vi "Main.vi"() -> ()   [LabVIEW 2019]
doc: "This template is for the Queued Message Handler design pattern.\n\nThe Event Handling Loop generates messages based on user interface actions.\n\nThe Message Handling Loop processes messages generated by the Event Handling Loop, or by other messages. The messages are string values, so new messages can be added easily to the Message Cases case structure in the Message Handling Loop. Each message cluster can also provide an optional value for Message Data, which is a variant that can be converted to whatever message-specific data is required."
uses:
  controls/UI Data.ctl
  support/Message Queue/Enqueue Message (Single).vi
  GlobalVI.vi
  <vilib>/Instr/_visa.llb/VISA Configure Serial Port (Instr).vi
  <vilib>/Utility/error.llb/Error Cluster From Error Code.vi
  <vilib>/httpClient/POSTBuffer.vi
  <vilib>/ErrorRing/Error Ring.xnode
  <vilib>/regexp/Match Regular Expression.xnode
  support/Message Queue/Message Queue.lvlib
  support/User Event - Stop/User Event - Stop.lvlib
  <vilib>/httpClient/LabVIEWHTTPClient.lvlib
panel:
  in  "disconnectSerial":bool
  out "f":T1(ring)
  out "current time":timestamp format="%<%X\n%x>T"
  in  "disconnectSerial":bool
  in  "Tab Control":T2(tab)
  in  "E-mail":string
  in  "Name":string
  in  "UID":string
  in  "RequestHTTPLogout":bool
  out "authorized":bool
  in  "Password":string
  in  "Login":string
  in  "RequestHTTPLogin":bool
  in  "DeleteEmploye":bool
  in  "OK Button 2":bool
  in  "NewEmployee":bool
  in  "Hire date (dd/mm/yyyy hh:mm:ss)":string
  in  "Hourly Payment ($)":dbl
  in  "UID":string
  in  "E-mail":string
  in  "Name":string
  in  "Role":u16(ring) items=["Admin 1", "Admin 2", "Worker 1", "Worker 2"]
  in  "Hire Date":string
  out "Hourly Rate":dbl
  in  "Name":string
  in  "Check In":string
  in  "UID":string
  out "Role":u16(ring) items=["Admin 1", "Admin 2", "Worker 1", "Worker 2"]
  in  "Check In":string
  out "Work Hours":dbl
  in  "Hire Date":string
  out "Hourly Rate":dbl
  in  "Name":string
  in  "Check Out":string
  in  "UID":string
  out "Role":u16(ring) items=["Admin 1", "Admin 2", "Worker 1", "Worker 2"]
  out "buffer":string
  in  "Communication Port":refnum<visa-resource-name>
  out "Display <Replace Me>":string
  in  "connect":bool
  in  "Exit":bool
  # "Read Employee Info"
  # "put your card in our RFID\nreader to fill this field"
  # "put your card in our RFID\nreader to fill this field"
  # "put your card in our RFID\nreader to fill this field"
  # "put your card in our RFID\nreader to fill this field"
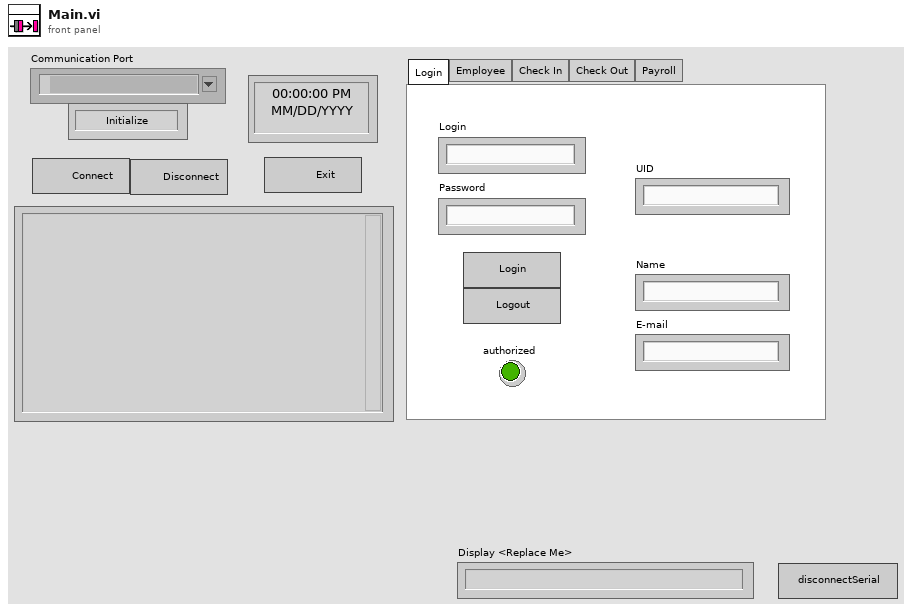
[diagram p1: front panel]
types:
  T1 = enum16{"Initialize", "Idle", "Connect", "Connected", "Disconnect", ""}
  T2 = enum32{"Login", "Employee", "Check In", "Check Out", "Payroll"}
  T3 = enum16{"Initialize", "Idle", "Connect", "Connected", "Disconnect"}
  T4 = typedef "UI Data.ctl" = cluster{"Boolean <Replace Me>":bool, "String <Replace Me>":string, "Numeric <Replace Me>":dbl, "Do Something Ref":refnum<vi>, "Do Something Else Ref":refnum<vi>, "Data Display Ref":refnum<vi>, "Exit Button Ref":refnum<vi>}
  T5 = typedef "LabVIEWHTTPClient.lvlib/ClientHandle.ctl" = refnum<k1>
  T6 = typedef "Message Queue.lvlib/All Message Queues.ctl" = cluster{"UI":refnum<queue>, "HTTP":refnum<queue>, "Serial":refnum<queue>}
  T7 = cluster{"name":string, "email":string, "uid":string, "hire_date":string, "hourly_rate":dbl, "job":cluster{"id":u8}}
  T8 = cluster{"id":u8, "checkIn":string, "checkOut":string, "work_hours":string, "employee":cluster{"id":u8, "name":string, "email":string, "uid":string, "hourly_rate":dbl, "hire_date":string, "job":cluster{"id":u8}, "createdAt":string}, "createdAt":string}
  T9 = cluster{"id":u8, "checkIn":string, "checkOut":string, "work_hours":dbl, "employee":cluster{"id":u8, "name":string, "email":string, "uid":string, "hourly_rate":dbl, "hire_date":string, "job":cluster{"id":u8}, "createdAt":string}, "createdAt":string}
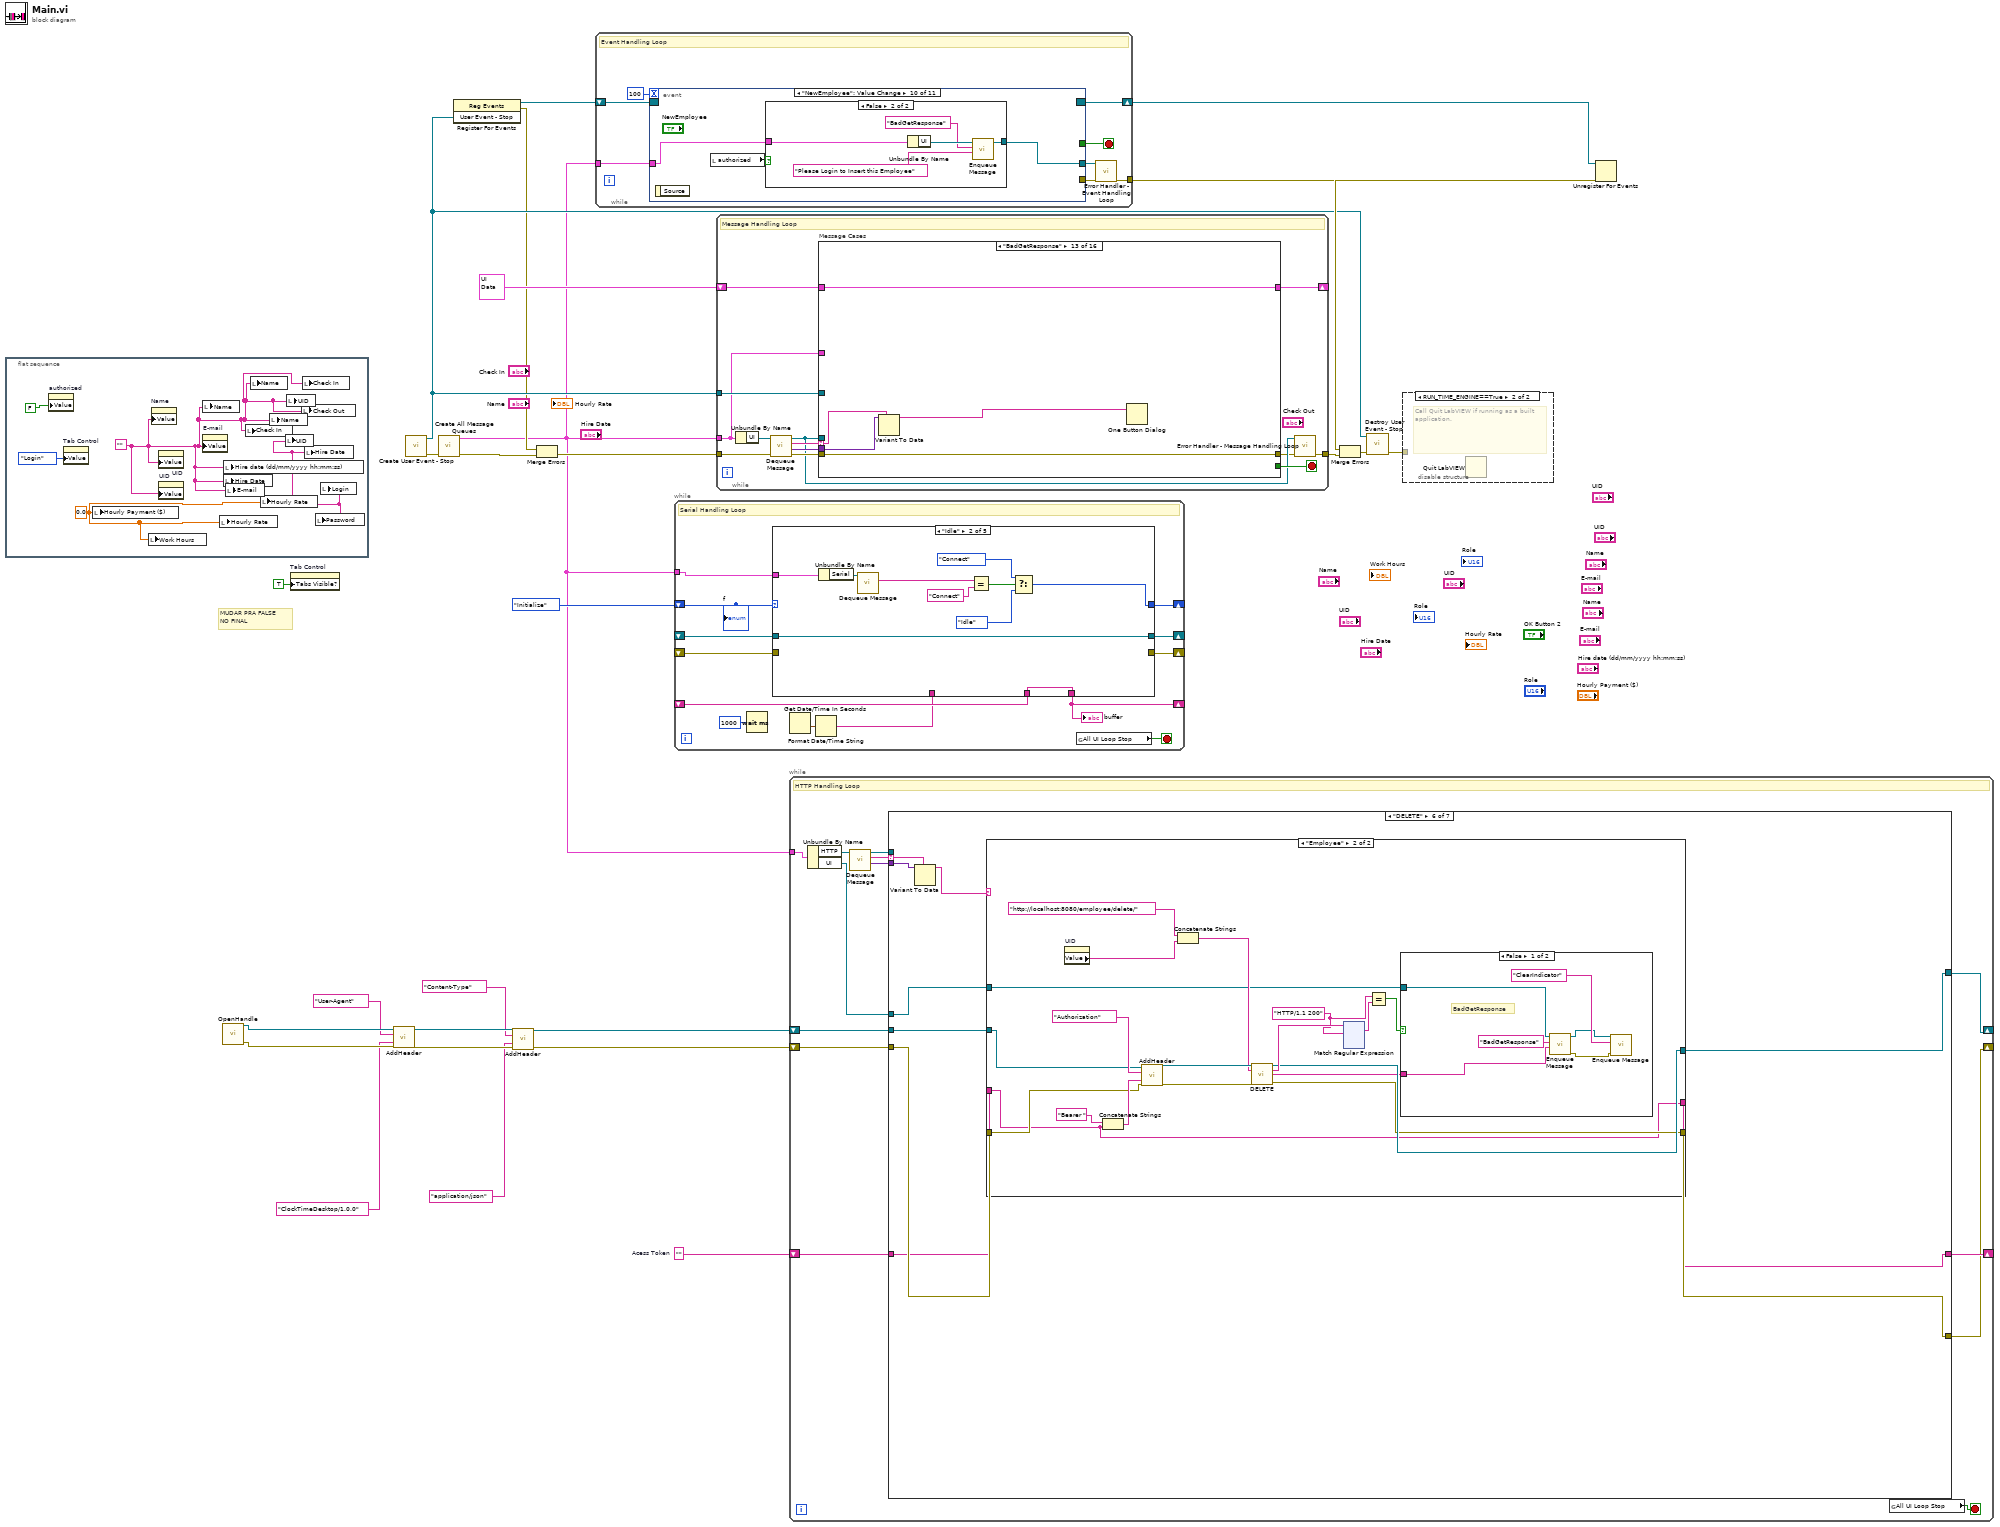
[diagram p0: block diagram]
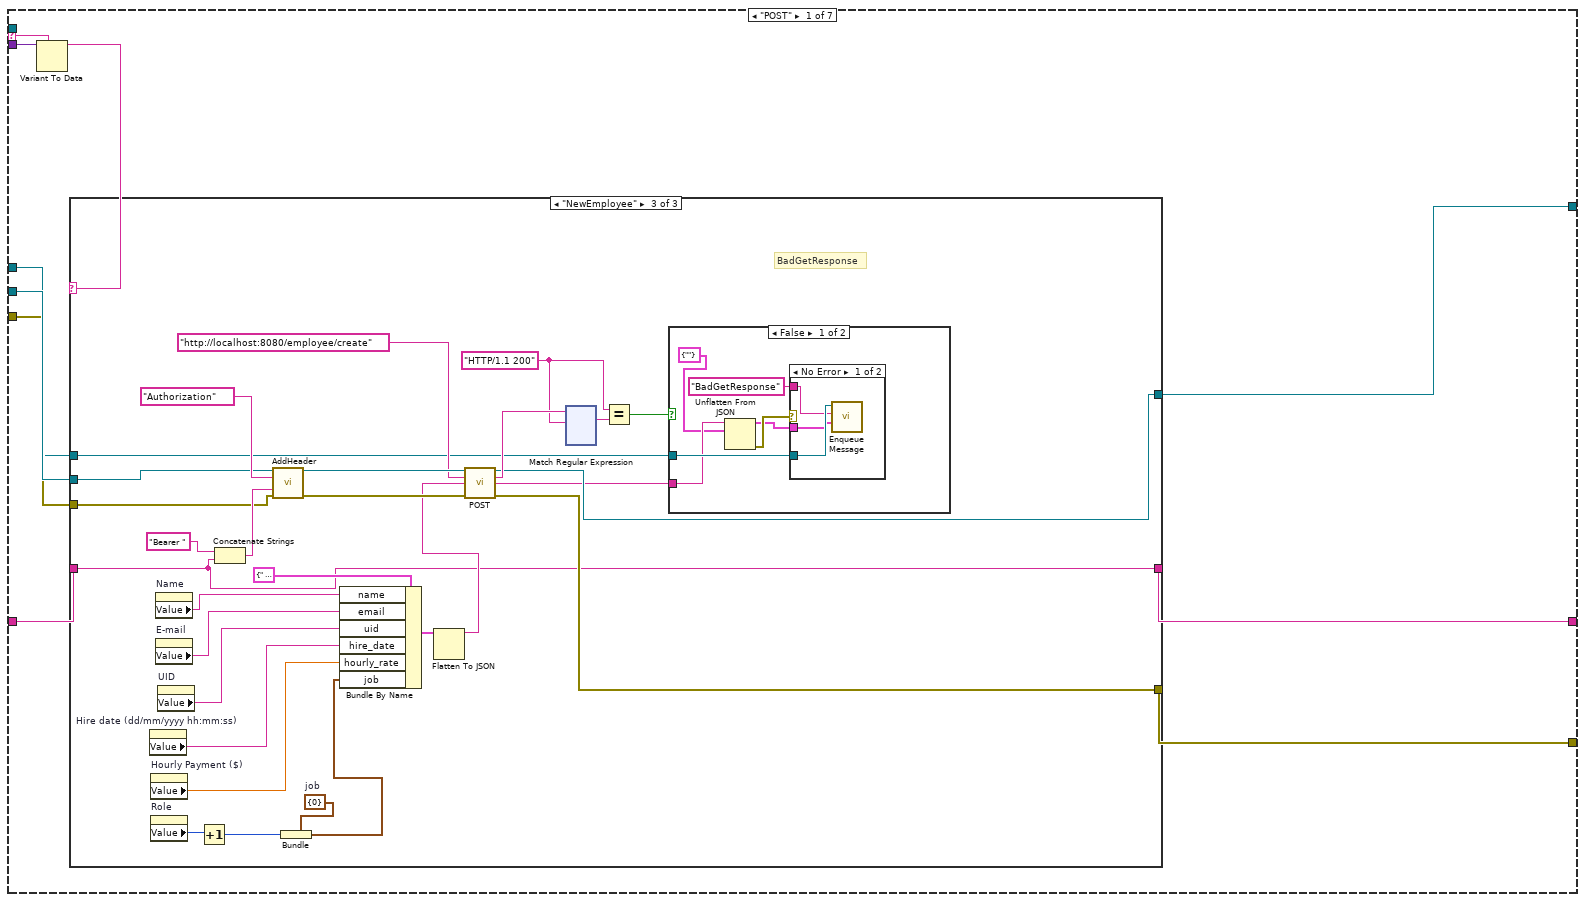
[diagram p2: hidden frame]
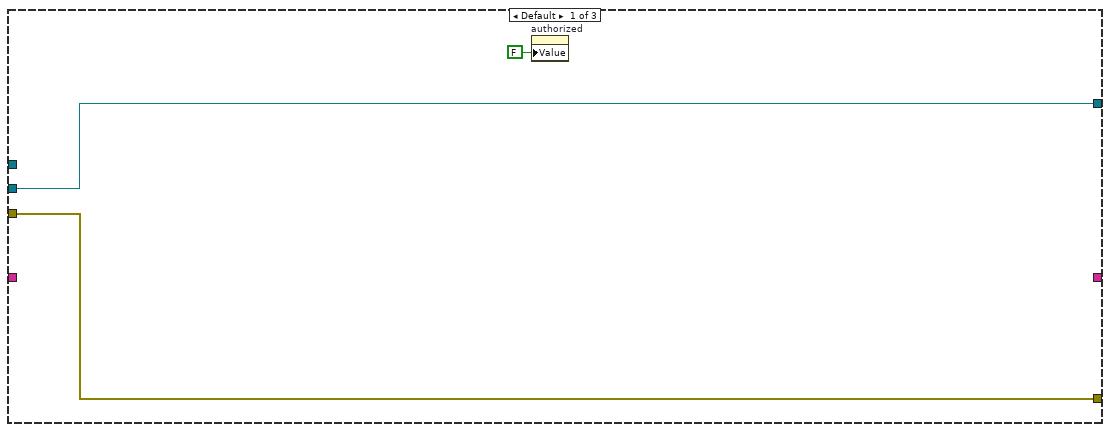
[diagram p3: hidden frame]
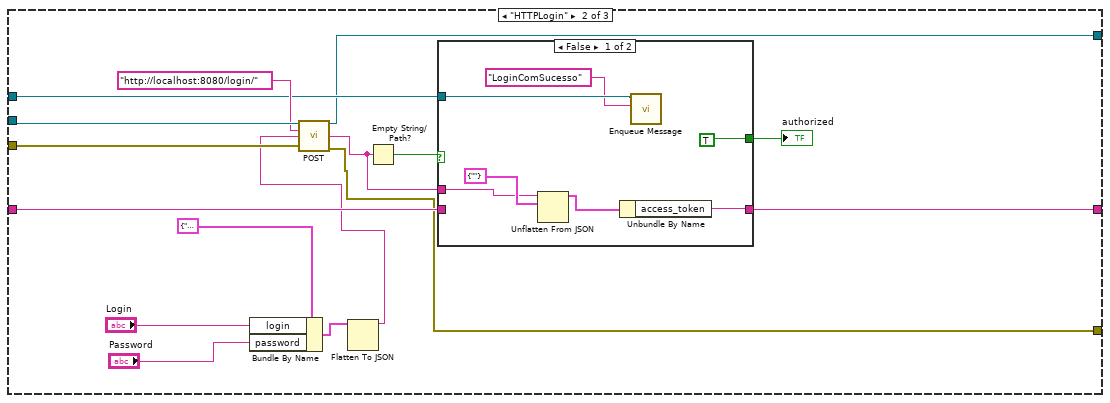
[diagram p4: hidden frame]
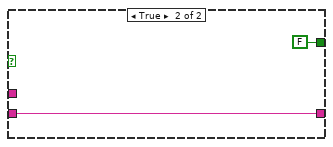
[diagram p5: hidden frame]
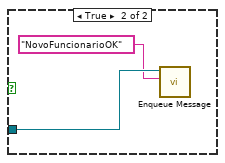
[diagram p7: hidden frame]
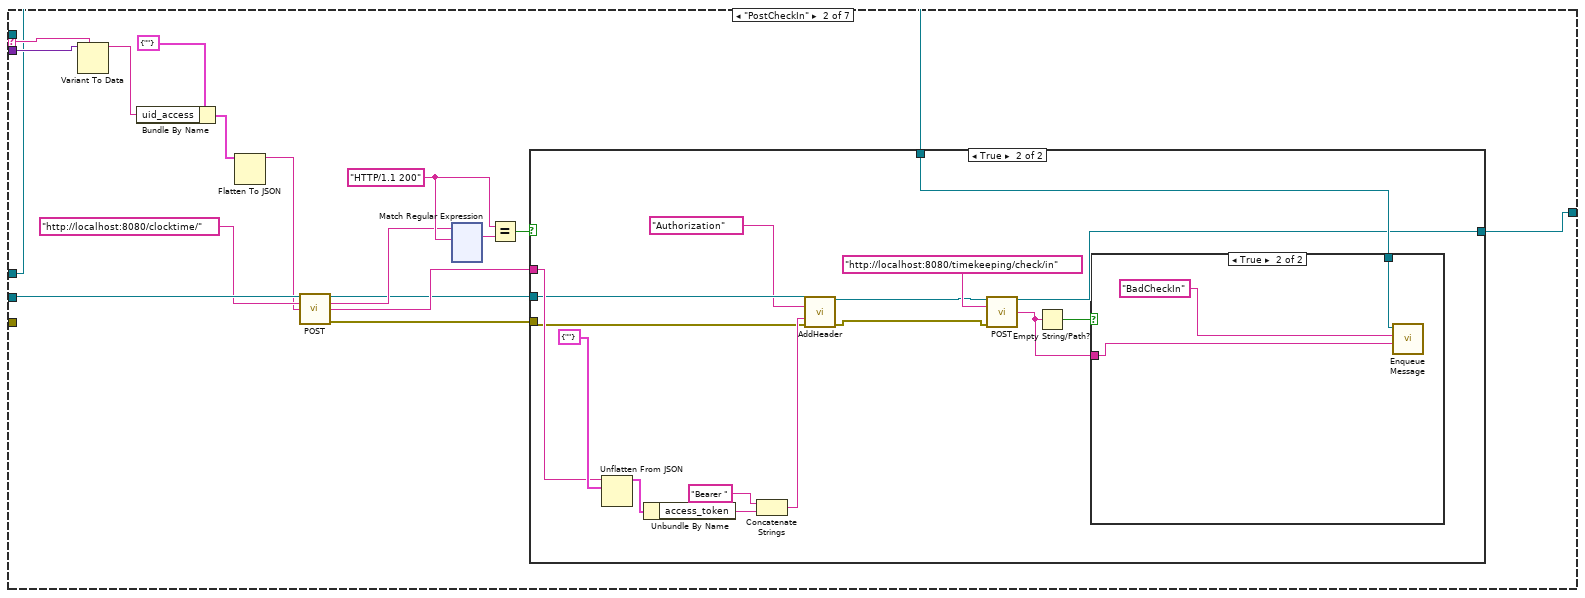
[diagram p8: hidden frame]
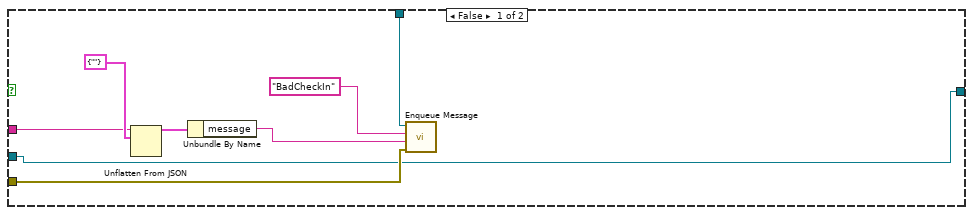
[diagram p9: hidden frame]
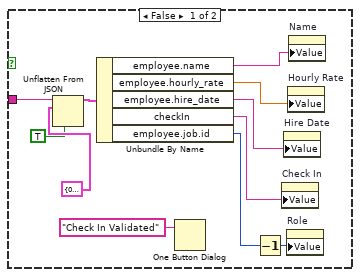
[diagram p10: hidden frame]
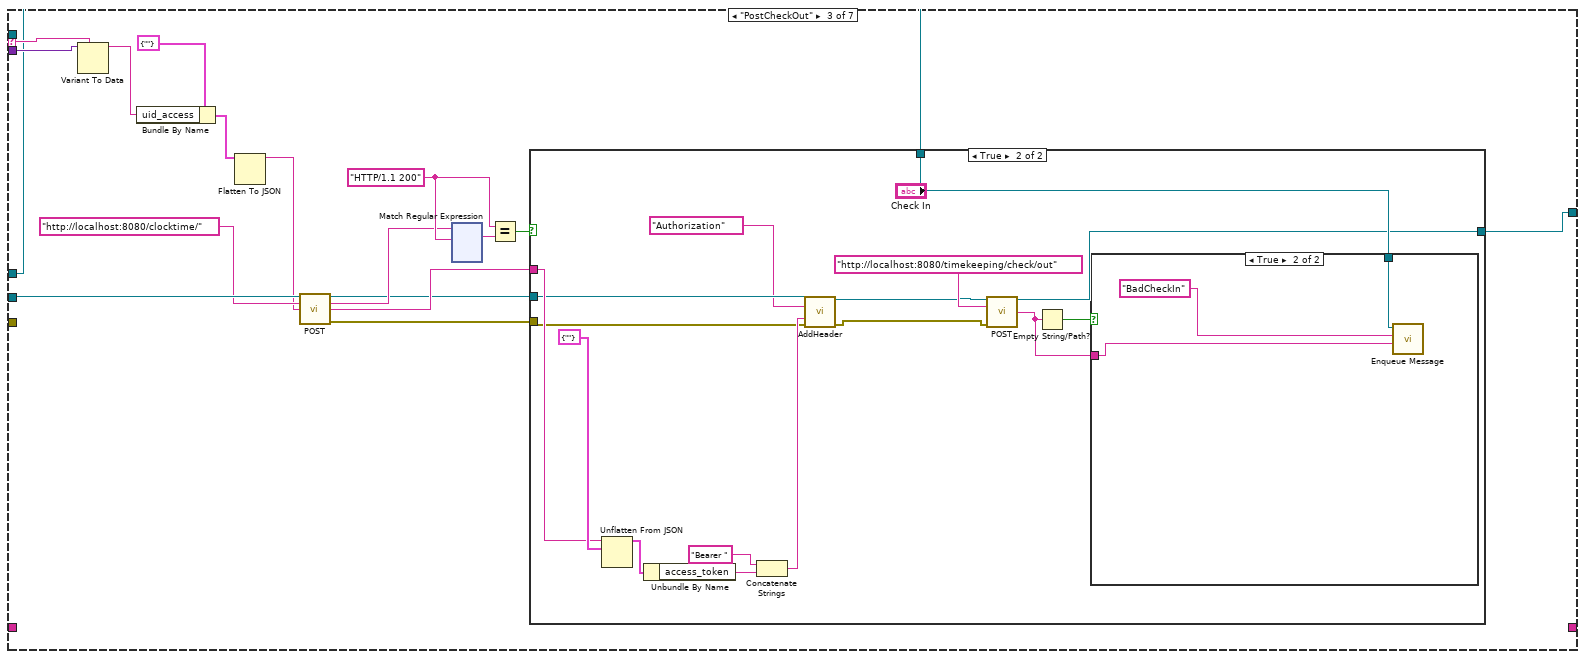
[diagram p11: hidden frame]
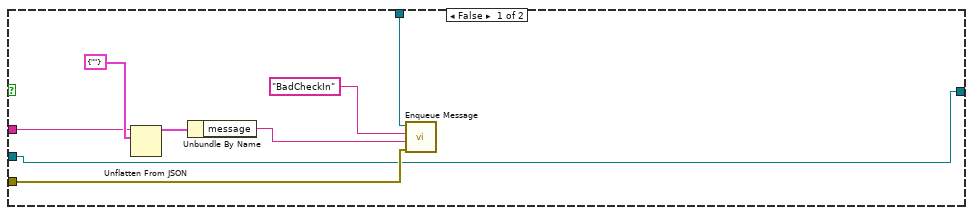
[diagram p12: hidden frame]
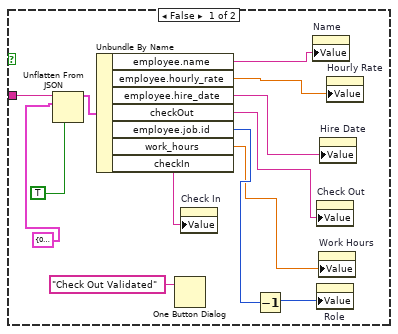
[diagram p13: hidden frame]
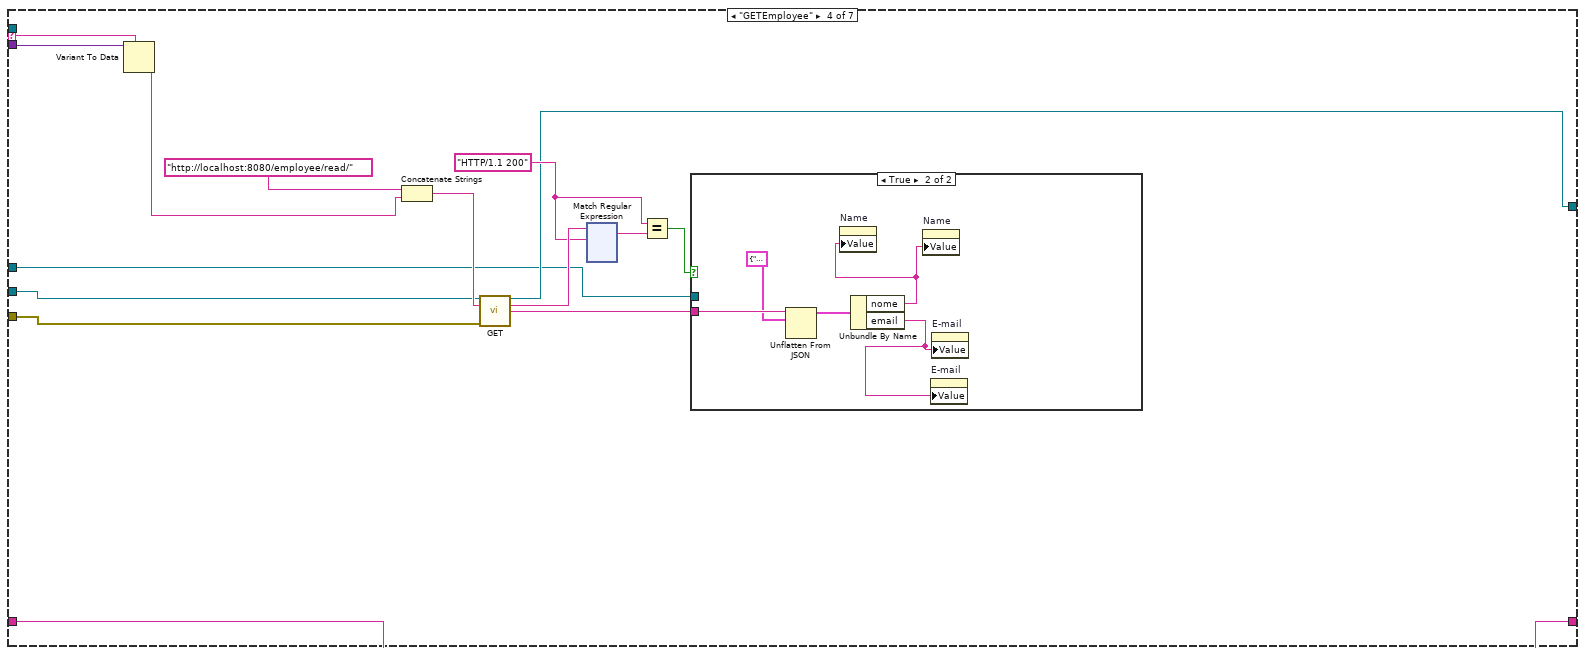
[diagram p14: hidden frame]
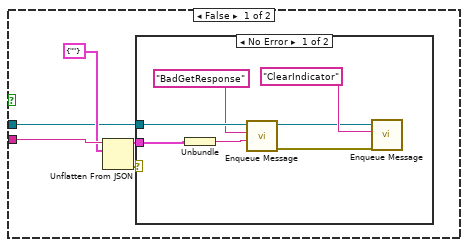
[diagram p15: hidden frame]
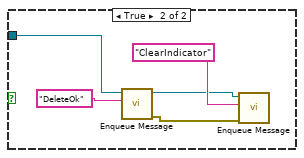
[diagram p19: hidden frame]
diagram:
  w12 = ""  # Acess Token
  # "MUDAR PRA FALSE \nNO FINAL"
  n1 = flat-sequence {
    frame #0 {
      w29 = 0.0 ("Hourly Payment ($)")
      w28 = ""
      n2 = property on="authorized" class="Bool (strict)"("Value"=FALSE ("authorized")) -> ()  [unwired: 2 in, 2 out]
      n3 = property on="Tab Control" class="TabCtl (strict)"("Value"=T2."Login" ("Tab Control")) -> ()  [unwired: 2 in, 2 out]
      n4 = local write "Hourly Payment ($)"(w29) -> ()
      n5 = local write "Work Hours"(w29) -> ()
      n6 = property on="Name" class="Str"("Value"=w28) -> ()  [unwired: 2 in, 2 out]
      n7 = property on="UID" class="Str"("Value"=w28) -> ()  [unwired: 2 in, 2 out]
      n8 = property on="UID" class="Str"("Value"=w28) -> ()  [unwired: 2 in, 2 out]
      n9 = local write "Name"(w28) -> ()
      n10 = property on="E-mail" class="Str"("Value"=w28) -> ()  [unwired: 2 in, 2 out]
      n11 = local write "Hourly Rate"(w29) -> ()
      n12 = local write "Hire date (dd/mm/yyyy hh:mm:ss)"(w28) -> ()
      n13 = local write "Hire Date"(w28) -> ()
      n14 = local write "E-mail"(w28) -> ()
      n15 = local write "Check In"(w28) -> ()
      n16 = local write "Name"(w28) -> ()
      n17 = local write "Hourly Rate"(w29) -> ()
      n18 = local write "Name"(w28) -> ()
      n19 = local write "UID"(w28) -> ()
      n20 = local write "UID"(w28) -> ()
      n21 = local write "Check Out"(w28) -> ()
      n22 = local write "Check In"(w28) -> ()
      n23 = local write "Hire Date"(w28) -> ()
      n24 = local write "Password"(w28) -> ()
      n25 = local write "Login"(w28) -> ()
    }
  }
  n26 = call <vilib>:"OpenHandle.vi"() -> ("client handle out"=w11:T5, "error out"=w9:errorcluster)  [unwired: 14 in]
  n27 = property on="Tab Control" class="TabCtl (strict)"("Tabs Visible?"=TRUE) -> ()  [unwired: 2 in, 2 out]
  n28 = call <vilib>:"AddHeader.vi"("client handle"=w11, "header"="User-Agent", "value"="ClockTimeDesktop/1.0.0", "error in (no error)"=w9) -> ("client handle out"=w10:T5, "error out"=w8:errorcluster)  [unwired: 10 in]
  n29 = call "Create User Event - Stop.vi"() -> ("error out"=w25:errorcluster, "User Event - Stop"=w17:refnum<user-event>)  [unwired: 10 in]
  n30 = call "Create All Message Queues.vi"("error in (no error)"=w25) -> ("error out"=w27:errorcluster, "Message Queues out"=w13:T6)  [unwired: 9 in]
  n31 = register-events(w17) -> (reference out=w18:refnum<event-registration>, error out=w15:errorcluster)  [unwired: 2 in]
  n32 = call <vilib>:"AddHeader.vi"("client handle"=w10, "header"="Content-Type", "value"="application/json", "error in (no error)"=w8) -> ("client handle out"=w7:T5, "error out"=w6:errorcluster)  [unwired: 10 in]
  n33 = Merge Errors(w15, w27) -> (w16:errorcluster)
  n34 = while {
    tunnel: w13 -> [w39]
    shift-right: [w37] -> w22
    shift-left: w18 -> [w38]
    tunnel: [w34] -> w19
    stop <- w35 stop-if-true
    # "Event Handling Loop"
    n35 = event shown="[9] \"NewEmployee\": Value Change" {
      selector: w38 -> [_ _ _ _ _ _ _ _ _ _ _]
      dyn-events: [_ _ _ _ _ _ _ _ _ _ _] -> w37
      timeout: 100 -> [_ _ _ _ _ _ _ _ _ _ _]
      tunnel: [_ _ _ _ _ _ _ TRUE ("Discard?") _ _ _] -> w35
      tunnel: w39 -> [w44 _ _ w52 w58 _ w62 _ w70 w75 w87]
      tunnel: [w42 _ _ w50 w57 _ w65 _ w71 _ w88] -> w36
      tunnel: [w40 _ _ w48 w53 _ w60 _ w72 w74 w89] -> w33
      event "connect": Value Change {
        n36 = event-data() -> ()  [unwired: 1 in, 1 out]
        n37 = Unbundle By Name(w44) -> ("Serial"=w41:refnum<queue>)
        n38 = call-poly "Enqueue Message.vi"("Message"="Connect", "Message Queue"=w41) -> ("error out"=w42:errorcluster, "dup Message Queue"=w40:refnum<queue>)  [unwired: 8 in]
      }
      event Timeout {
        n39 = event-data() -> ()  [unwired: 1 in, 1 out]
        n40 = Get Date/Time In Seconds() -> (seconds since 1Jan1904=→"current time":timestamp)
      }
      event "disconnectSerial": Value Change {
        n41 = event-data() -> ()  [unwired: 1 in, 1 out]
        n42 = property on="disconnectSerial" class="Bool (strict)"("Value"=TRUE ("disconnectSerial")) -> ()  [unwired: 2 in, 2 out]
      }
      event "RequestHTTPLogin": Value Change {
        n43 = event-data() -> ()  [unwired: 1 in, 1 out]
        n44 = Unbundle By Name(w52) -> ("HTTP"=w49:refnum<queue>)
        n45 = call-poly "Enqueue Message.vi"("Message Data"="HTTPLogin" ("Message"), "Message"="POST", "Message Queue"=w49) -> ("error out"=w50:errorcluster, "dup Message Queue"=w48:refnum<queue>)  [unwired: 7 in]
      }
      event Panel Close? {
        # "Send the 'Confirm Quit' message if the user closes the panel of the VI. Discard the event so the 'Confirm Quit' message has a chance to run."
        n46 = event-data() -> ()  [unwired: 1 in, 1 out]
        n47 = Unbundle By Name(w58) -> ("UI"=w54:refnum<queue>)
        n48 = call-poly "Enqueue Message.vi"("Priority Message? (F)"=TRUE, "Message"="Confirm Quit", "Message Queue"=w54) -> ("error out"=w57:errorcluster, "dup Message Queue"=w53:refnum<queue>)  [unwired: 7 in]
        n49 = event-data("Discard?"=TRUE) -> ()  [unwired: 1 in, 1 out]
      }
      event Application Instance Close {
        # "#CodeRecommended - When a project closes, all VIs within that project are aborted and leave memory. However, any code placed in this event frame is guaranteed to run to completion, so add any cleanup code that absolutely must happen here."
        n50 = event-data() -> ()  [unwired: 1 in, 1 out]
      }
      event "Exit": Value Change {
        n51 = event-data() -> ()  [unwired: 1 in, 1 out]
        n52 = Unbundle By Name(w62) -> ("UI"=w61:refnum<queue>)
        n53 = call-poly "Enqueue Message.vi"("Priority Message? (F)"=TRUE, "Message"="Exit", "Message Queue"=w61) -> ("error out"=w65:errorcluster, "dup Message Queue"=w60:refnum<queue>)  [unwired: 7 in]
      }
      event User Event {
        # "The Message Handling Loop processed an \"Exit\" message, which fired this event to stop the Event Handling Loop."
        n54 = event-data() -> ()  [unwired: 1 in, 1 out]
        n55 = local write "Display <Replace Me>"("\"Exit\" button pressed" ("VI Stopped")) -> ()
      }
      event "RequestHTTPLogout": Value Change {
        n56 = event-data() -> ()  [unwired: 1 in, 1 out]
        n57 = Unbundle By Name(w70) -> ("HTTP"=w69:refnum<queue>)
        n58 = call-poly "Enqueue Message.vi"("Message"="POST", "Message Queue"=w69) -> ("error out"=w71:errorcluster, "dup Message Queue"=w72:refnum<queue>)  [unwired: 8 in]
      }
      event "NewEmployee": Value Change {
        n59 = event-data() -> ()  [unwired: 1 in, 1 out]
        n60 = local read "authorized"() -> (w73:bool)
        n61 = case shown="False" w73 {
          tunnel: w75 -> [w80 w85]
          tunnel: [w76 w81] -> w74
          frame True {
            n62 = Unbundle By Name(w80) -> ("HTTP"=w79:refnum<queue>)
            n63 = call-poly "Enqueue Message.vi"("Message Data"="NewEmployee" ("Message"), "Message"="POST", "Message Queue"=w79) -> ("dup Message Queue"=w76:refnum<queue>)  [unwired: 7 in, 1 out]
          }
          frame False {
            n64 = Unbundle By Name(w85) -> ("UI"=w84:refnum<queue>)
            n65 = call-poly "Enqueue Message.vi"("Message Data"="Please Login to Insert this Employee" ("Message"), "Message"="BadGetResponse", "Message Queue"=w84) -> ("dup Message Queue"=w81:refnum<queue>)  [unwired: 7 in, 1 out]
          }
        }
      }
      event "DeleteEmploye": Value Change {
        n66 = event-data() -> ()  [unwired: 1 in, 1 out]
        n67 = local read "authorized"() -> (w86:bool)
        n68 = case shown="False" w86 {
          tunnel: [w95 w101] -> w89
          tunnel: [w94 w100] -> w88
          tunnel: w87 -> [w93 w99]
          frame True {
            n69 = Unbundle By Name(w93) -> ("HTTP"=w92:refnum<queue>)
            n70 = call-poly "Enqueue Message.vi"("Message Data"="Employee" ("Message"), "Message"="DELETE", "Message Queue"=w92) -> ("error out"=w94:errorcluster, "dup Message Queue"=w95:refnum<queue>)  [unwired: 7 in]
          }
          frame False {
            n71 = Unbundle By Name(w99) -> ("UI"=w98:refnum<queue>)
            n72 = call-poly "Enqueue Message.vi"("Message Data"="Please Login to delete this employee" ("Message"), "Message"="BadGetResponse", "Message Queue"=w98) -> ("error out"=w100:errorcluster, "dup Message Queue"=w101:refnum<queue>)  [unwired: 7 in]
          }
        }
      }
    }
    n73 = call "Error Handler - Event Handling Loop.vi"("error in (no error)"=w36, "Message Queue"=w33) -> ("dup error in"=w34:errorcluster)  [unwired: 8 in, 1 out]
  }
  n74 = while {
    tunnel: w13 -> [w111]
    shift-right: [w112] -> _
    shift-left: T3."Initialize" -> [w113]
    shift-right: [w110] -> _
    shift-left: _ -> [w108]
    shift-right: [w109] -> _
    shift-left: _ -> [w107]
    shift-right: [w105] -> _
    shift-left: _ -> [w106]
    stop <- w114 stop-if-true
    # "Serial Handling Loop"
    n75 = Wait (ms)(milliseconds to wait=u32 1000) -> ()  [unwired: 1 out]
    n76 = Get Date/Time In Seconds() -> (seconds since 1Jan1904=w104:timestamp)
    n77 = Format Date/Time String(seconds (now)=w104) -> (date/time string=w103:string)  [unwired: 2 in]
    n78 = case shown="\"Idle\"" w113 {
      tunnel: [T1."Idle" w118 w133 w142 _] -> w112
      tunnel: w111 -> [_ w124 _ w145 _]
      tunnel: [_ w117 w135 w143 _] -> w110
      tunnel: [_ _ w134 w144 w180] -> w109
      tunnel: w108 -> [_ w117 _ w149 w182]
      tunnel: w107 -> [_ _ _ w141 w181]
      tunnel: w106 -> [_ w116 w127 w139 w172]
      tunnel: [_ w116 w130 w138 w177] -> w105
      tunnel: w103 -> [_ _ w129 w137 w175]
      frame "Initialize", Default {
      }
      frame "Idle" {
        n79 = Unbundle By Name(w124) -> ("Serial"=w125:refnum<queue>)
        n80 = call "Dequeue Message.vi"("Message Queue"=w125) -> ("Message"=w123:string)  [unwired: 7 in, 3 out]
        n81 = Equal?(x=w123, y="Connect") -> (x = y?=w121:bool)
        n82 = Select(t=T1."Connect", s=w121, f=T1."Idle") -> (s? t:f=w118:T1)
      }
      frame "Connect" {
        n83 = call-poly "VISA Configure Serial Port"("VISA resource name"="Communication Port") -> ("VISA resource name out"=w135:refnum<visa-resource-name>, "error out"=w134:errorcluster)  [unwired: 13 in]
        n84 = Concatenate Strings("\r\n", w129, " - Connect" ("string"), w127) -> (w130:string)
        n85 = Select(t=T1."Idle" ("f"), s=w134, f=T1."Connected") -> (s? t:f=w133:T1)
      }
      frame "Connected" {
        n86 = property class="Instr"(reference=w149, error in=w141) -> (reference out=w147:refnum<visa-resource-name>, error out=w146:errorcluster, "Bytes at Port"=w140:u32)
        n87 = Greater Than 0?(x=w140) -> (x > 0?=w148:bool)
        n88 = case shown="True" w148 {
          tunnel: w147 -> [w157 w171]
          tunnel: w146 -> [w156 w170]
          tunnel: w145 -> [_ w169]
          tunnel: [w156 w166] -> w144
          tunnel: [w157 w165] -> w143
          tunnel: [w150 T1."Connected"] -> w142
          tunnel: w140 -> [_ w163]
          tunnel: w139 -> [w154 w158]
          tunnel: [w154 w162] -> w138
          tunnel: w137 -> [_ w161]
          frame False {
            w152 = T1."Disconnect"
            n89 = Select(t=w152, s=w156, f=T1."Connected") -> (s? t:f=w151:T1)
            n90 = Select(t=w152, s="disconnectSerial", f=w151) -> (s? t:f=w150:T1)
          }
          frame True {
            n91 = VISA Read(VISA resource name=w171, byte count=w163, error in (no error)=w170) -> (VISA resource name out=w165:refnum<visa-resource-name>, read buffer=w160:string, error out=w166:errorcluster)  [unwired: 1 out]
            n92 = Unbundle By Name(w169) -> ("UI"=w168:refnum<queue>)
            n93 = call-poly "Enqueue Message.vi"("Message Data"=w160, "Message"="SerialData", "Message Queue"=w168) -> ()  [unwired: 7 in, 2 out]
            n94 = Concatenate Strings(w161, " - " ("string"), w160, w158) -> (w162:string)
          }
        }
      }
      frame "Disconnect" {
        n95 = VISA Clear(VISA resource name=w182, error in (no error)=w181) -> (VISA resource name out=w179:refnum<visa-resource-name>, error out=w178:errorcluster)
        n96 = VISA Close(VISA resource name=w179, error in (no error)=w178) -> (error out=w180:errorcluster)
        n97 = property on="disconnectSerial" class="Bool (strict)"("Value"=FALSE ("disconnectSerial")) -> ()  [unwired: 2 in, 2 out]
        n98 = Concatenate Strings("\r\n", w175, " - Disconnected" ("string"), w172) -> (w177:string)
      }
    }
    "buffer" <- w105
    n99 = global read "GlobalVI.vi" "All UI Loop Stop"() -> (w114:bool)
    "f" <- w113
  }
  n100 = while {
    tunnel: w13 -> [w183]
    shift-right: [w194] -> _
    shift-left: T4 {"Boolean <Replace Me>"=FALSE, "String <Replace Me>"="", "Numeric <Replace Me>"=0.0, "Do Something Ref"=refnum, "Do Something Else Ref"=refnum, "Data Display Ref"=refnum, "Exit Button Ref"=refnum} ("Data Cluster") -> [w195]
    tunnel: w17 -> [w192]
    tunnel: w16 -> [w191]
    tunnel: [w186] -> w26
    stop <- w193 stop-if-true
    # "Message Handling Loop"
    n101 = Unbundle By Name(w183) -> ("UI"=w184:refnum<queue>)
    n102 = call "Dequeue Message.vi"("error in (no error)"=w191, "Message Queue"=w184) -> ("error out"=w190:errorcluster, "Message Data"=w188:variant, "Message"=w189:string, "dup Message Queue"=w187:refnum<queue>)  [unwired: 6 in]
    n103 = case "Message Cases" shown="\"BadGetResponse\"" w189 {
      selector: w189 -> [_ _ _ _ _ _ _ _ w263 w284 _ _ w303 _ _ w315]
      tunnel: w187 -> [w197 w209 w216 _ _ w237 _ w256 _ _ _ _ _ _ _ _]
      tunnel: w190 -> [w205 w211 w218 w225 w234 w241 w244 w249 w266 w289 w297 w300 w305 w310 w312 _]
      tunnel: [w206 w212 w219 w226 w228 w239 w242 w252 w266 w289 w297 w300 w305 w310 w312 w316] -> w185
      tunnel: w195 -> [w204 w213 w220 w227 w233 w240 w243 w255 w265 w288 w296 w299 w304 w309 w314 w317]
      tunnel: [w203 w213 w220 w227 w233 w240 w243 w255 w265 w288 w296 w299 w304 w309 w314 w317] -> w194
      tunnel: [_ _ _ _ _ _ _ TRUE _ _ _ _ _ _ _ _] -> w193
      tunnel: w188 -> [_ _ _ w224 w232 _ _ w246 w264 w285 _ _ w302 _ _ _]
      tunnel: w192 -> [_ _ _ _ _ _ _ w251 _ _ _ _ _ _ _ _]
      tunnel: w183 -> [_ _ _ _ _ _ _ _ w257 _ _ _ _ _ _ _]
      frame "Initialize" {
        w196 = "ClearIndicator" ("Initial Message")
        # "Initialize - All initialization work should take place in this message, since other loops can potentially enqueue messages that execute immediately after this one."
        n104 = control-ref of="connect"() -> (w202:refnum<vi>)
        n105 = control-ref of="RequestHTTPLogin"() -> (w201:refnum<vi>)
        n106 = control-ref of="Exit"() -> (w199:refnum<vi>)
        n107 = control-ref of="Display <Replace Me>"() -> (w200:refnum<vi>)
        n108 = Bundle By Name(cluster=w204, "Do Something Ref"=w202, "Do Something Else Ref"=w201, "Data Display Ref"=w200, "Exit Button Ref"=w199, "String <Replace Me>"=w196) -> (w203:T4)
        n109 = call-poly "Enqueue Message.vi"("error in (no error)"=w205, "Message Data"=w196, "Message"="Update Display", "Message Queue"=w197) -> ("error out"=w206:errorcluster)  [unwired: 6 in, 1 out]
      }
      frame "Something" {
        # "Send string to \"Update Display\" message"
        # "#CodeNeeded - Perform whatever actions correspond to the \"Something\" message."
        # "Something - Replace this message with functionality for your own application."
        n110 = call-poly "Enqueue Message.vi"("error in (no error)"=w211, "Message Data"="\"Do Something\" button pressed" ("\"Do Something\" button pressed"), "Message"="Update Display", "Message Queue"=w209) -> ("error out"=w210:errorcluster)  [unwired: 6 in, 1 out]
        n111 = Merge Errors(w210) -> (w212:errorcluster)
      }
      frame "Something Else" {
        # "Send string to \"Update Display\" message"
        # "#CodeNeeded - Perform whatever actions correspond to the \"Something Else\" message."
        # "Something Else - Replace this message with functionality for your own application."
        n112 = call-poly "Enqueue Message.vi"("error in (no error)"=w218, "Message Data"="\"Do Something Else\" button pressed" ("\"Do Something Else\" button pressed"), "Message"="Update Display", "Message Queue"=w216) -> ("error out"=w217:errorcluster)  [unwired: 6 in, 1 out]
        n113 = Merge Errors(w217) -> (w219:errorcluster)
      }
      frame "Update Display" {
        # "#CodeRecommended - If you wish to decouple the Message Handling Loop from your user interface, consider creating User Events (like the \"Stop\" event in this VI) to message the Event Handling Loop whenever the user interface needs updating."
        # "Update Display - Convert the message data to a string to display in the Data Display indicator."
        n114 = Variant To Data(error in=w225, type="", Variant=w224) -> (data=→"Display <Replace Me>":string, error out=w222:errorcluster)
        n115 = Merge Errors(w222) -> (w226:errorcluster)
      }
      frame "Error" {
        # "#CodeRecommended - If you ever change the name of this \"Error\" message, you'll need to update the name in the Check Loop Error.vi as well."
        # "#CodeRecommended - Consider creating a system for logging errors in some way. These errors are for notification purposes only. Handling of specific errors should be performed in the message frames that generated the error."
        # "Error - Display an error dialog. This message is sent by the \"Error Handler\" VIs at the end of other loops in this application."
        n116 = Variant To Data(error in=w234, type=errorcluster {"status"=FALSE, "code"=0, "source"=""} ("error constant"), Variant=w232) -> (data=w230:errorcluster, error out=w229:errorcluster)
        n117 = call <vilib>:"Simple Error Handler.vi"("error in (no error)"=w230) -> ()  [unwired: 4 in, 5 out]
        n118 = Merge Errors(w229) -> (w228:errorcluster)
      }
      frame "Confirm Quit" {
        # "#CodeNeeded - If you want to provide an \"Are you sure\" dialog (or some other notification) before the application exits, place that code here. This message is typically sent from a Panel Close? event."
        # "Confirm Quit - Message that can confirm whether or not the user wants to exit the application."
        n119 = call-poly "Enqueue Message.vi"("Priority Message? (F)"=TRUE, "error in (no error)"=w241, "Message"="Exit", "Message Queue"=w237) -> ("error out"=w238:errorcluster)  [unwired: 6 in, 1 out]
        n120 = Merge Errors(w238) -> (w239:errorcluster)
      }
      frame "---Copy This Frame---" {
        # "Duplicate this frame when creating new messages.  Change this comment in the duplicated frame to describe this message."
        n121 = Merge Errors(w244) -> (w242:errorcluster)
      }
      frame "Exit" {
        # "Stop the VI"
        # "Release the message queue reference"
        # "#CodeNeeded - Add any required cleanup code here. Note that if 'Exit' was called as a result of an error, an error dialog will be displayed. Add any custom error handling for an 'Exit' condition here as well."
        # "Exit - Exit the application."
        n122 = Variant To Data(type=errorcluster {"status"=FALSE, "code"=0, "source"=""} ("error constant"), Variant=w246) -> (data=w247:errorcluster)  [unwired: 1 in, 1 out]
        n123 = call <vilib>:"Simple Error Handler.vi"("error in (no error)"=w247) -> ()  [unwired: 4 in, 5 out]
        n124 = call "Fire User Event - Stop.vi"("User Event - Stop"=w251) -> ("error out"=w250:errorcluster)  [unwired: 10 in]
        n125 = Release Queue(queue=w256, error in (no error)=w249) -> (error out=w253:errorcluster)  [unwired: 1 in, 2 out]
        n126 = global write "GlobalVI.vi" "All UI Loop Stop"(TRUE ("All UI Loop Stop")) -> ()
        n127 = Merge Errors(w250, w253) -> (w252:errorcluster)
      }
      frame "SerialData" {
        # "quando vier dado SERIAL"
        n128 = Variant To Data(type=w263, Variant=w264) -> (data=w262:string)  [unwired: 1 in, 1 out]
        n129 = Match Pattern(string=w262, regular expression=":") -> (after substring=w260:string)  [unwired: 1 in, 3 out]
        n130 = call <vilib>:"Trim Whitespace.vi"("string"=w260) -> ("trimmed string"=w258:string)  [unwired: 1 in]
        n131 = Empty String/Path?(string/path=w258) -> (empty?=w259:bool)
        n132 = case shown="False" w259 {
          tunnel: w258 -> [w267 _]
          tunnel: w257 -> [w269 _]
          frame False {
            n133 = case shown="\"Check Out\"" "Tab Control" {
              tunnel: w269 -> [_ w273 w277 w281]
              tunnel: w267 -> [_ w270 w274 w278]
              frame Default {
              }
              frame "Login", "Employee" {
                n134 = Unbundle By Name(w273) -> ("HTTP"=w272:refnum<queue>)
                n135 = property on="UID" class="Str"("Value"=w270) -> ()  [unwired: 2 in, 2 out]
                n136 = property on="UID" class="Str"("Value"=w270) -> ()  [unwired: 2 in, 2 out]
                n137 = call-poly "Enqueue Message.vi"("Message Data"=w270, "Message"="GETEmployee", "Message Queue"=w272) -> ()  [unwired: 7 in, 2 out]
              }
              frame "Check In" {
                n138 = Unbundle By Name(w277) -> ("HTTP"=w276:refnum<queue>)
                n139 = property on="UID" class="Str"("Value"=w274) -> ()  [unwired: 2 in, 2 out]
                n140 = call-poly "Enqueue Message.vi"("Message Data"=w274, "Message"="PostCheckIn", "Message Queue"=w276) -> ()  [unwired: 7 in, 2 out]
              }
              frame "Check Out" {
                n141 = Unbundle By Name(w281) -> ("HTTP"=w280:refnum<queue>)
                n142 = property on="UID" class="Str"("Value"=w278) -> ()  [unwired: 2 in, 2 out]
                n143 = call-poly "Enqueue Message.vi"("Message Data"=w278, "Message"="PostCheckOut", "Message Queue"=w280) -> ()  [unwired: 7 in, 2 out]
              }
            }
          }
          frame True {
          }
        }
      }
      frame "BadCheckIn" {
        n144 = Variant To Data(type=w284, Variant=w285) -> (data=w283:string)  [unwired: 1 in, 1 out]
        n145 = Concatenate Strings("Invalid UID! Can`t validate your Work. Please Contact our Suport\nsuport@sup.ck.nt" ("message"), "\r\n", w283) -> (w282:string)
        n146 = One Button Dialog(message=w282) -> ()  [unwired: 1 in, 1 out]
      }
      frame "NovoFuncionarioOK" {
        n147 = Get Date/Time In Seconds() -> (seconds since 1Jan1904=w295:timestamp)
        n148 = Get Date/Time String(seconds (now)=w295) -> (date string=w293:string, time string=w292:string)  [unwired: 2 in]
        n149 = Get Date/Time In Seconds() -> ()  [unwired: 1 out]
        n150 = call <vilib>:"Space Constant.vi"() -> ("String"=w290:string)
        n151 = Concatenate Strings("New Employee insert successfully |  ", w293, w290, w292) -> (w291:string)
        n152 = One Button Dialog(message=w291) -> ()  [unwired: 1 in, 1 out]
      }
      frame "LoginComSucesso" {
        n153 = property on="Tab Control" class="TabCtl (strict)"("Tabs Visible?"=TRUE) -> ()  [unwired: 2 in, 2 out]
      }
      frame "BadGetResponse" {
        n154 = Variant To Data(type=w303, Variant=w302) -> (data=w301:string)  [unwired: 1 in, 1 out]
        n155 = One Button Dialog(message=w301) -> ()  [unwired: 1 in, 1 out]
      }
      frame "ClearIndicator" {
        w306 = ""
        n156 = local write "Hourly Payment ($)"(0.0 ("Hourly Payment ($)")) -> ()
        n157 = local write "Hire date (dd/mm/yyyy hh:mm:ss)"(w306) -> ()
        n158 = local write "Name"(w306) -> ()
        n159 = local write "E-mail"(w306) -> ()
        n160 = local write "E-mail"(w306) -> ()
        n161 = local write "Name"(w306) -> ()
        n162 = local write "UID"(w306) -> ()
        n163 = property on="Tab Control" class="TabCtl (strict)"() -> ("Value"=w307:T2)  [unwired: 2 in, 2 out]
        n164 = case shown="\"Employee\"" w307 {
          tunnel: w306 -> [w311 _]
          frame Default {
            n165 = local write "UID"(w311) -> ()
          }
          frame "Employee" {
          }
        }
        n166 = property on="Login" class="Str"("Value"=w306) -> ()  [unwired: 2 in, 2 out]
        n167 = property on="Password" class="Str"("Value"=w306) -> ()  [unwired: 2 in, 2 out]
      }
      frame "DeleteOk" {
        n168 = One Button Dialog(message="The current employee was deleted ") -> ()  [unwired: 1 in, 1 out]
      }
      frame Default {
        # "'Default' case only runs if there is a message that isn't defined in any of the other cases.  Output a programming error."
        n169 = xnode "Error Ring"("parameter 0"=w315) -> ("error out"=w316:errorcluster)
      }
    }
    n170 = call "Error Handler - Message Handling Loop.vi"("error in (no error)"=w185, "Message Queue"=w187) -> ("dup error in"=w186:errorcluster)  [unwired: 8 in, 1 out]
  }
  n171 = while {
    tunnel: w13 -> [w336]
    shift-right: [w328] -> _
    shift-left: w12 -> [w329]
    shift-right: [w326] -> _
    shift-left: w7 -> [w331]
    shift-right: [w325] -> _
    shift-left: w6 -> [w330]
    stop <- w337 stop-if-true
    # "HTTP Handling Loop"
    n172 = Unbundle By Name(w336) -> ("HTTP"=w333:refnum<queue>, "UI"=w327:refnum<queue>)
    n173 = call "Dequeue Message.vi"("Message Queue"=w333) -> ("Message Data"=w332:variant, "Message"=w335:string, "dup Message Queue"=w334:refnum<queue>)  [unwired: 7 in, 1 out]
    n174 = case shown="\"DELETE\"" w335 {
      selector: w335 -> [w346 w545 w714 w883 _ w1027 _]
      tunnel: w334 -> [_ _ _ _ _ _ _]
      tunnel: w332 -> [w347 w546 w715 w884 _ w1028 _]
      tunnel: w331 -> [w344 w544 w713 w879 w1017 w1024 w1177]
      tunnel: w330 -> [w343 _ _ w878 w1016 w1022 w1176]
      tunnel: w329 -> [w342 _ _ w872 w1018 w1020 _]
      tunnel: [w341 _ _ w872 w1018 w1021 _] -> w328
      tunnel: w327 -> [w340 w534 w703 w870 _ w1019 _]
      tunnel: [w339 w530 w699 w871 w1017 w1025 w1177] -> w326
      tunnel: [w338 _ _ _ w1016 w1023 w1176] -> w325
      frame "POST" {
        n175 = Variant To Data(type=w346, Variant=w347) -> (data=w345:string)  [unwired: 1 in, 1 out]
        n176 = case shown="\"NewEmployee\"" w345 {
          tunnel: w344 -> [w350 w366 w400]
          tunnel: w343 -> [w349 w365 w401]
          tunnel: w342 -> [_ w362 w377]
          tunnel: [_ w360 w377] -> w341
          tunnel: w340 -> [_ w359 w380]
          tunnel: [w350 w352 w379] -> w339
          tunnel: [w349 w351 w378] -> w338
          frame Default {
            n177 = property on="authorized" class="Bool (strict)"("Value"=FALSE ("authorized")) -> ()  [unwired: 2 in, 2 out]
          }
          frame "HTTPLogin" {
            n178 = Bundle By Name(cluster=cluster{"login":string, "password":string} {"login"="", "password"=""} ("anything"), "login"="Login", "password"="Password") -> (w355:cluster{"login":string, "password":string})
            n179 = Flatten To JSON(anything=w355) -> (JSON string=w354:string)  [unwired: 2 in, 1 out]
            n180 = call-poly <vilib>:"POST.vi"("client handle"=w366, "url"="http://localhost:8080/login/", "buffer"=w354, "error in (no error)"=w365) -> ("client handle out"=w352:T5, "body"=w361:string, "error out"=w351:errorcluster)  [unwired: 8 in, 1 out]
            n181 = Empty String/Path?(string/path=w361) -> (empty?=w363:bool)
            n182 = case shown="False" w363 {
              tunnel: w362 -> [_ w375]
              tunnel: w361 -> [w372 _]
              tunnel: [w370 w375] -> w360
              tunnel: w359 -> [w369 _]
              tunnel: [TRUE FALSE] -> w353
              frame False {
                n183 = Unflatten From JSON(JSON string=w372, type and defaults=cluster{"access_token":string} {"access_token"=""}) -> (value=w371:cluster{"access_token":string})  [unwired: 5 in, 1 out]
                n184 = Unbundle By Name(w371) -> ("access_token"=w370:string)
                n185 = call-poly "Enqueue Message.vi"("Message"="LoginComSucesso", "Message Queue"=w369) -> ()  [unwired: 8 in, 2 out]
              }
              frame True {
              }
            }
            "authorized" <- w353
          }
          frame "NewEmployee" {
            w382 = "HTTP/1.1 200" ("regular expression")
            w386 = cluster{"id":u8} {"id"=0}  # job
            # "BadGetResponse"
            n186 = property on="Hire date (dd/mm/yyyy hh:mm:ss)" class="Str"() -> ("Value"=w390:string)  [unwired: 2 in, 2 out]
            n187 = property on="Hourly Payment ($)" class="DigNum (strict)"() -> ("Value"=w389:dbl)  [unwired: 2 in, 2 out]
            n188 = property on="Role" class="Ring (strict)"() -> ("Value"=w388:u16)  [unwired: 2 in, 2 out]
            n189 = property on="Name" class="Str"() -> ("Value"=w393:string)  [unwired: 2 in, 2 out]
            n190 = property on="E-mail" class="Str"() -> ("Value"=w392:string)  [unwired: 2 in, 2 out]
            n191 = property on="UID" class="Str"() -> ("Value"=w391:string)  [unwired: 2 in, 2 out]
            n192 = Increment(x=w388) -> (x+1=w385:u16)
            n193 = Concatenate Strings("Bearer ", w377) -> (w402:string)
            n194 = call <vilib>:"AddHeader.vi"("client handle"=w400, "header"="Authorization", "value"=w402, "error in (no error)"=w401) -> ("client handle out"=w399:T5, "error out"=w398:errorcluster)  [unwired: 10 in]
            n195 = Bundle(cluster=w386, "id"=w385) -> (w387:cluster{"id":u8})
            n196 = Bundle By Name(cluster=T7 {"name"=" ", "email"=" ", "uid"=" ", "hire_date"=" ", "hourly_rate"=0.0, "job"={"id"=0}}, "name"=w393, "email"=w392, "uid"=w391, "hire_date"=w390, "hourly_rate"=w389, "job"=w387) -> (w395:T7)
            n197 = Flatten To JSON(anything=w395) -> (JSON string=w394:string)  [unwired: 2 in, 1 out]
            n198 = call-poly <vilib>:"POST.vi"("client handle"=w399, "url"="http://localhost:8080/employee/create", "buffer"=w394, "error in (no error)"=w398) -> ("client handle out"=w379:T5, "headers"=w384:string, "body"=w376:string, "error out"=w378:errorcluster)  [unwired: 8 in]
            n199 = xnode "Match Regular Expression"("input string"=w384, "regular expression"=w382) -> ("whole match"=w383:string)  [unwired: 4 in, 4 out]
            n200 = Equal?(x=w382, y=w383) -> (x = y?=w381:bool)
            n201 = case shown="False" w381 {
              tunnel: w380 -> [w410 w415]
              tunnel: w376 -> [w408 _]
              frame False {
                n202 = Unflatten From JSON(JSON string=w408, type and defaults=cluster{"message":string} {"message"=""}) -> (value=w405:cluster{"message":string}, error out=w406:errorcluster)  [unwired: 5 in]
                n203 = case shown="No Error" w406 {
                  tunnel: w410 -> [w413 _]
                  tunnel: "BadGetResponse" ("Message") -> [w412 _]
                  tunnel: w405 -> [w411 _]
                  frame No Error {
                    n204 = call-poly "Enqueue Message.vi"("Message Data"=w411, "Message"=w412, "Message Queue"=w413) -> ()  [unwired: 7 in, 2 out]
                  }
                  frame Error {
                  }
                }
              }
              frame True {
                n205 = call-poly "Enqueue Message.vi"("Message"="NovoFuncionarioOK", "Message Queue"=w415) -> ()  [unwired: 8 in, 2 out]
              }
            }
          }
        }
      }
      frame "PostCheckIn" {
        w537 = "HTTP/1.1 200" ("regular expression")
        n206 = Variant To Data(type=w545, Variant=w546) -> (data=w541:string)  [unwired: 1 in, 1 out]
        n207 = Bundle By Name(cluster=cluster{"uid_access":string} {"uid_access"=""}, "uid_access"=w541) -> (w540:cluster{"uid_access":string})
        n208 = Flatten To JSON(anything=w540) -> (JSON string=w539:string)  [unwired: 2 in, 1 out]
        n209 = call-poly <vilib>:"POST.vi"("client handle"=w544, "url"="http://localhost:8080/clocktime/", "buffer"=w539) -> ("client handle out"=w531:T5, "headers"=w536:string, "body"=w532:string, "error out"=w533:errorcluster)  [unwired: 9 in]
        n210 = xnode "Match Regular Expression"("input string"=w536, "regular expression"=w537) -> ("whole match"=w538:string)  [unwired: 4 in, 4 out]
        n211 = Equal?(x=w537, y=w538) -> (x = y?=w535:bool)
        n212 = case shown="True" w535 {
          tunnel: w534 -> [w554 w557]
          tunnel: w533 -> [w552 w559]
          tunnel: w532 -> [w550 w568]
          tunnel: w531 -> [w547 w567]
          tunnel: [w547 w555] -> w530
          frame False {
            n213 = Unflatten From JSON(JSON string=w550, type and defaults=cluster{"message":string} {"message"=""}) -> (value=w549:cluster{"message":string})  [unwired: 5 in, 1 out]
            n214 = Unbundle By Name(w549) -> ("message"=w548:string)
            n215 = call-poly "Enqueue Message.vi"("error in (no error)"=w552, "Message Data"=w548, "Message"="BadCheckIn", "Message Queue"=w554) -> ()  [unwired: 6 in, 2 out]
          }
          frame True {
            n216 = Unflatten From JSON(JSON string=w568, type and defaults=cluster{"access_token":string} {"access_token"=""}) -> (value=w563:cluster{"access_token":string})  [unwired: 5 in, 1 out]
            n217 = Unbundle By Name(w563) -> ("access_token"=w561:string)
            n218 = Concatenate Strings("Bearer ", w561) -> (w564:string)
            n219 = call <vilib>:"AddHeader.vi"("client handle"=w567, "header"="Authorization", "value"=w564, "error in (no error)"=w559) -> ("client handle out"=w566:T5, "error out"=w560:errorcluster)  [unwired: 10 in]
            n220 = call-poly <vilib>:"POST.vi"("client handle"=w566, "url"="http://localhost:8080/timekeeping/check/in", "error in (no error)"=w560) -> ("client handle out"=w555:T5, "body"=w556:string)  [unwired: 9 in, 2 out]
            n221 = Empty String/Path?(string/path=w556) -> (empty?=w558:bool)
            n222 = case shown="True" w558 {
              tunnel: w557 -> [_ w583]
              tunnel: w556 -> [w581 w582]
              frame False {
                n223 = Unflatten From JSON(JSON string=w581, type and defaults=T8 {"id"=0, "checkIn"="", "checkOut"="", "work_hours"="", "employee"={"id"=0, "name"="", "email"="", "uid"="", "hourly_rate"=0.0, "hire_date"="", "job"={"id"=0}, "createdAt"=""}, "createdAt"=""}, default null elements? (F)=TRUE) -> (value=w580:T8)  [unwired: 4 in, 1 out]
                n224 = Unbundle By Name(w580) -> ("employee.name"=w579:string, "employee.hourly_rate"=w578:dbl, "employee.hire_date"=w577:string, "checkIn"=w576:string, "employee.job.id"=w574:u8)
                n225 = One Button Dialog(message="Check In Validated") -> ()  [unwired: 1 in, 1 out]
                n226 = Decrement(x=w574) -> (x-1=w575:u8)
                n227 = property on="Check In" class="Str"("Value"=w576) -> ()  [unwired: 2 in, 2 out]
                n228 = property on="Hire Date" class="Str"("Value"=w577) -> ()  [unwired: 2 in, 2 out]
                n229 = property on="Role" class="Ring (strict)"("Value"=w575) -> ()  [unwired: 2 in, 2 out]
                n230 = property on="Hourly Rate" class="DigNum (strict)"("Value"=w578) -> ()  [unwired: 2 in, 2 out]
                n231 = property on="Name" class="Str"("Value"=w579) -> ()  [unwired: 2 in, 2 out]
              }
              frame True {
                n232 = call-poly "Enqueue Message.vi"("Message Data"=w582, "Message"="BadCheckIn", "Message Queue"=w583) -> ()  [unwired: 7 in, 2 out]
              }
            }
          }
        }
      }
      frame "PostCheckOut" {
        w706 = "HTTP/1.1 200" ("regular expression")
        n233 = Variant To Data(type=w714, Variant=w715) -> (data=w710:string)  [unwired: 1 in, 1 out]
        n234 = Bundle By Name(cluster=cluster{"uid_access":string} {"uid_access"=""}, "uid_access"=w710) -> (w709:cluster{"uid_access":string})
        n235 = Flatten To JSON(anything=w709) -> (JSON string=w708:string)  [unwired: 2 in, 1 out]
        n236 = call-poly <vilib>:"POST.vi"("client handle"=w713, "url"="http://localhost:8080/clocktime/", "buffer"=w708) -> ("client handle out"=w700:T5, "headers"=w705:string, "body"=w701:string, "error out"=w702:errorcluster)  [unwired: 9 in]
        n237 = xnode "Match Regular Expression"("input string"=w705, "regular expression"=w706) -> ("whole match"=w707:string)  [unwired: 4 in, 4 out]
        n238 = Equal?(x=w706, y=w707) -> (x = y?=w704:bool)
        n239 = case shown="True" w704 {
          tunnel: w703 -> [w723 w726]
          tunnel: w702 -> [w721 w728]
          tunnel: w701 -> [w719 w737]
          tunnel: w700 -> [w716 w736]
          tunnel: [w716 w724] -> w699
          frame False {
            n240 = Unflatten From JSON(JSON string=w719, type and defaults=cluster{"message":string} {"message"=""}) -> (value=w718:cluster{"message":string})  [unwired: 5 in, 1 out]
            n241 = Unbundle By Name(w718) -> ("message"=w717:string)
            n242 = call-poly "Enqueue Message.vi"("error in (no error)"=w721, "Message Data"=w717, "Message"="BadCheckIn", "Message Queue"=w723) -> ()  [unwired: 6 in, 2 out]
          }
          frame True {
            n243 = Unflatten From JSON(JSON string=w737, type and defaults=cluster{"access_token":string} {"access_token"=""}) -> (value=w732:cluster{"access_token":string})  [unwired: 5 in, 1 out]
            n244 = Unbundle By Name(w732) -> ("access_token"=w730:string)
            n245 = Concatenate Strings("Bearer ", w730) -> (w733:string)
            n246 = call <vilib>:"AddHeader.vi"("client handle"=w736, "header"="Authorization", "value"=w733, "error in (no error)"=w728) -> ("client handle out"=w735:T5, "error out"=w729:errorcluster)  [unwired: 10 in]
            n247 = call-poly <vilib>:"POST.vi"("client handle"=w735, "url"="http://localhost:8080/timekeeping/check/out", "error in (no error)"=w729) -> ("client handle out"=w724:T5, "body"=w725:string)  [unwired: 9 in, 2 out]
            n248 = Empty String/Path?(string/path=w725) -> (empty?=w727:bool)
            n249 = case shown="True" w727 {
              tunnel: w726 -> [_ w754]
              tunnel: w725 -> [w752 w753]
              frame False {
                n250 = Unflatten From JSON(JSON string=w752, type and defaults=T9 {"id"=0, "checkIn"="", "checkOut"="", "work_hours"=0.0, "employee"={"id"=0, "name"="", "email"="", "uid"="", "hourly_rate"=0.0, "hire_date"="", "job"={"id"=0}, "createdAt"=""}, "createdAt"=""}, default null elements? (F)=TRUE) -> (value=w751:T9)  [unwired: 4 in, 1 out]
                n251 = Unbundle By Name(w751) -> ("employee.name"=w747:string, "employee.hourly_rate"=w746:dbl, "employee.hire_date"=w741:string, "checkOut"=w742:string, "employee.job.id"=w750:u8, "work_hours"=w745:dbl, "checkIn"=w740:string)
                n252 = One Button Dialog(message="Check Out Validated") -> ()  [unwired: 1 in, 1 out]
                n253 = property on="Check In" class="Str"("Value"=w740) -> ()  [unwired: 2 in, 2 out]
                n254 = Decrement(x=w750) -> (x-1=w743:u8)
                n255 = property on="Name" class="Str"("Value"=w747) -> ()  [unwired: 2 in, 2 out]
                n256 = property on="Check Out" class="Str"("Value"=w742) -> ()  [unwired: 2 in, 2 out]
                n257 = property on="Role" class="Ring (strict)"("Value"=w743) -> ()  [unwired: 2 in, 2 out]
                n258 = property on="Work Hours" class="DigNum (strict)"("Value"=w745) -> ()  [unwired: 2 in, 2 out]
                n259 = property on="Hire Date" class="Str"("Value"=w741) -> ()  [unwired: 2 in, 2 out]
                n260 = property on="Hourly Rate" class="DigNum (strict)"("Value"=w746) -> ()  [unwired: 2 in, 2 out]
              }
              frame True {
                n261 = call-poly "Enqueue Message.vi"("Message Data"=w753, "Message"="BadCheckIn", "Message Queue"=w754) -> ()  [unwired: 7 in, 2 out]
              }
            }
          }
        }
      }
      frame "GETEmployee" {
        w874 = "HTTP/1.1 200" ("regular expression")
        n262 = Variant To Data(type=w883, Variant=w884) -> (data=w881:string)  [unwired: 1 in, 1 out]
        n263 = Concatenate Strings("http://localhost:8080/employee/read/", w881) -> (w880:string)
        n264 = call <vilib>:"GET.vi"("client handle"=w879, "url"=w880, "error in (no error)"=w878) -> ("client handle out"=w871:T5, "headers"=w876:string, "body"=w877:string)  [unwired: 9 in, 1 out]
        n265 = xnode "Match Regular Expression"("input string"=w876, "regular expression"=w874) -> ("whole match"=w875:string)  [unwired: 4 in, 4 out]
        n266 = Equal?(x=w874, y=w875) -> (x = y?=w873:bool)
        n267 = case shown="True" w873 {
          tunnel: w877 -> [w889 w901]
          tunnel: w870 -> [w885 _]
          frame False {
            n268 = Unflatten From JSON(JSON string=w889, type and defaults=cluster{"message":string} {"message"=""}) -> (value=w886:cluster{"message":string}, error out=w887:errorcluster)  [unwired: 5 in]
            n269 = case shown="No Error" w887 {
              tunnel: w886 -> [w896 _]
              tunnel: w885 -> [w894 _]
              frame No Error {
                n270 = Unbundle(w896) -> ("message"=w895:string)
                n271 = call-poly "Enqueue Message.vi"("Message Data"=w895, "Message"="BadGetResponse", "Message Queue"=w894) -> ("error out"=w892:errorcluster, "dup Message Queue"=w890:refnum<queue>)  [unwired: 7 in]
                n272 = call-poly "Enqueue Message.vi"("error in (no error)"=w892, "Message"="ClearIndicator", "Message Queue"=w890) -> ()  [unwired: 7 in, 2 out]
              }
              frame Error {
              }
            }
          }
          frame True {
            n273 = Unflatten From JSON(JSON string=w901, type and defaults=cluster{"nome":string, "email":string} {"nome"="", "email"=""}) -> (value=w899:cluster{"nome":string, "email":string})  [unwired: 5 in, 1 out]
            n274 = Unbundle By Name(w899) -> ("nome"=w898:string, "email"=w897:string)
            n275 = property on="Name" class="Str"("Value"=w898) -> ()  [unwired: 2 in, 2 out]
            n276 = property on="Name" class="Str"("Value"=w898) -> ()  [unwired: 2 in, 2 out]
            n277 = property on="E-mail" class="Str"("Value"=w897) -> ()  [unwired: 2 in, 2 out]
            n278 = property on="E-mail" class="Str"("Value"=w897) -> ()  [unwired: 2 in, 2 out]
          }
        }
      }
      frame "PUT" {
      }
      frame "DELETE" {
        n279 = Variant To Data(type=w1027, Variant=w1028) -> (data=w1026:string)  [unwired: 1 in, 1 out]
        n280 = case shown="\"Employee\"" w1026 {
          tunnel: [w1031 w1035] -> w1025
          tunnel: w1024 -> [w1031 w1044]
          tunnel: [w1030 w1034] -> w1023
          tunnel: w1022 -> [w1030 w1045]
          tunnel: [w1029 w1033] -> w1021
          tunnel: w1020 -> [w1029 w1033]
          tunnel: w1019 -> [_ w1036]
          frame Default {
          }
          frame "Employee" {
            w1038 = "HTTP/1.1 200" ("regular expression")
            n281 = property on="UID" class="Str"() -> ("Value"=w1050:string)  [unwired: 2 in, 2 out]
            n282 = Concatenate Strings("Bearer ", w1033) -> (w1046:string)
            n283 = call <vilib>:"AddHeader.vi"("client handle"=w1044, "header"="Authorization", "value"=w1046, "error in (no error)"=w1045) -> ("client handle out"=w1043:T5, "error out"=w1042:errorcluster)  [unwired: 10 in]
            n284 = Concatenate Strings("http://localhost:8080/employee/delete/", w1050) -> (w1041:string)
            n285 = call <vilib>:"DELETE.vi"("client handle"=w1043, "url"=w1041, "error in (no error)"=w1042) -> ("client handle out"=w1035:T5, "headers"=w1040:string, "body"=w1032:string, "error out"=w1034:errorcluster)  [unwired: 9 in]
            n286 = xnode "Match Regular Expression"("input string"=w1040, "regular expression"=w1038) -> ("whole match"=w1039:string)  [unwired: 4 in, 4 out]
            n287 = Equal?(x=w1038, y=w1039) -> (x = y?=w1037:bool)
            n288 = case shown="False" w1037 {
              tunnel: w1036 -> [w1056 w1061]
              tunnel: w1032 -> [w1054 _]
              frame False {
                # "BadGetResponse"
                n289 = call-poly "Enqueue Message.vi"("Message Data"=w1054, "Message"="BadGetResponse", "Message Queue"=w1056) -> ("error out"=w1052:errorcluster, "dup Message Queue"=w1051:refnum<queue>)  [unwired: 7 in]
                n290 = call-poly "Enqueue Message.vi"("error in (no error)"=w1052, "Message"="ClearIndicator", "Message Queue"=w1051) -> ()  [unwired: 7 in, 2 out]
              }
              frame True {
                n291 = call-poly "Enqueue Message.vi"("Message"="DeleteOk", "Message Queue"=w1061) -> ("error out"=w1057:errorcluster, "dup Message Queue"=w1058:refnum<queue>)  [unwired: 8 in]
                n292 = call-poly "Enqueue Message.vi"("error in (no error)"=w1057, "Message"="ClearIndicator", "Message Queue"=w1058) -> ()  [unwired: 7 in, 2 out]
              }
            }
          }
        }
      }
      frame Default {
      }
    }
    n293 = global read "GlobalVI.vi" "All UI Loop Stop"() -> (w337:bool)
  }
  n294 = Unregister For Events(event registration refnum=w22, error in=w19) -> (error out=w23:errorcluster)
  n295 = Merge Errors(w23, w26) -> (w24:errorcluster)
  n296 = call "Destroy User Event - Stop.vi"("error in (no error)"=w24, "User Event - Stop"=w17) -> ("error out"=w20:errorcluster)  [unwired: 9 in]
  n297 = disable-structure shown="RUN_TIME_ENGINE==True" {
    disable-tunnel: w20 -> [_ _]
    frame condition #0 (active) {
    }
    frame condition #1 {
      # "Call Quit LabVIEW if running as a built application."
      n298 = Quit LabVIEW() -> ()  [unwired: 1 in]
    }
  }
